vi "Point To Row.vi"(8 "error in (no error)":errorcluster, 10 "Point":T1, 11 "ListBox in":refnum<class "ListBox.lvclass">) -> (0 "error out":errorcluster, 1 "Row":i32, 2 "In Bounds?":bool, 3 "ListBox out":refnum<class "ListBox.lvclass">, 4 "In Symbol?":bool)   [LabVIEW 2015, in "ListBox.lvclass"]
doc: "Converts a pixel coordinate to a row in the coordinates of the control. This method also returns whether the point is inside the bounds of the content rectangle and whether the point is within the custom symbol of the cell.\n\nQControl Class wrapper around the <b>ListBox : Point to Row Method</b>.\n<b> </b> <b> </b>\n©2016 Q Software Innovations, LLC (QSI)\nwritten by Quentin Alldredge\nproduced in LabVIEW 2015\n\nsupport@qsoftwareinnovations.com\nwww.qsoftwareinnovations.com\n\nAll rights reserved.\n\nRedistribution and use in source and binary forms, with or without modification, are permitted provided that the following conditions are met:\n\n * Redistributions of source code must retain the above copyright notice, this list of conditions and the following disclaimer.\n * Redistributions in binary form must reproduce the above copyright notice, this list of conditions and the following disclaimer in the documentation and/or other materials provided with the distribution.\n * Neither the name of Q Software Innovations, LLC. nor the names of its contributors may be used to endorse or promote products derived from this software without specific prior written permission.\n\nTHIS SOFTWARE IS PROVIDED BY THE COPYRIGHT HOLDERS AND CONTRIBUTORS \"AS IS\" AND ANY EXPRESS OR IMPLIED WARRANTIES, INCLUDING, BUT NOT LIMITED TO, THE IMPLIED WARRANTIES OF MERCHANTABILITY AND FITNESS FOR A PARTICULAR PURPOSE ARE DISCLAIMED. IN NO EVENT SHALL THE COPYRIGHT OWNER OR CONTRIBUTORS BE LIABLE FOR ANY DIRECT, INDIRECT, INCIDENTAL, SPECIAL, EXEMPLARY, OR CONSEQUENTIAL DAMAGES (INCLUDING, BUT NOT LIMITED TO, PROCUREMENT OF SUBSTITUTE GOODS OR SERVICES; LOSS OF USE, DATA, OR PROFITS; OR BUSINESS INTERRUPTION) HOWEVER CAUSED AND ON ANY THEORY OF LIABILITY, WHETHER IN CONTRACT, STRICT LIABILITY, OR TORT (INCLUDING NEGLIGENCE OR OTHERWISE) ARISING IN ANY WAY OUT OF THE USE OF THIS SOFTWARE, EVEN IF ADVISED OF THE POSSIBILITY OF SUCH DAMAGE."
uses:
  ListBox.lvclass
  <vilib>/Utility/miscctls.llb/LVPositionTypeDef.ctl
  ListBox.lvclass/ListBox.ctl
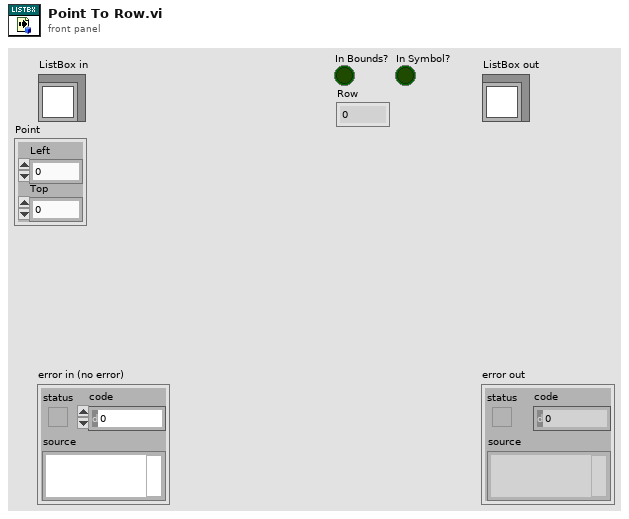
[diagram p1: front panel]
types:
  T1 = typedef "LVPositionTypeDef.ctl" = cluster{"Left":i32, "Top":i32}
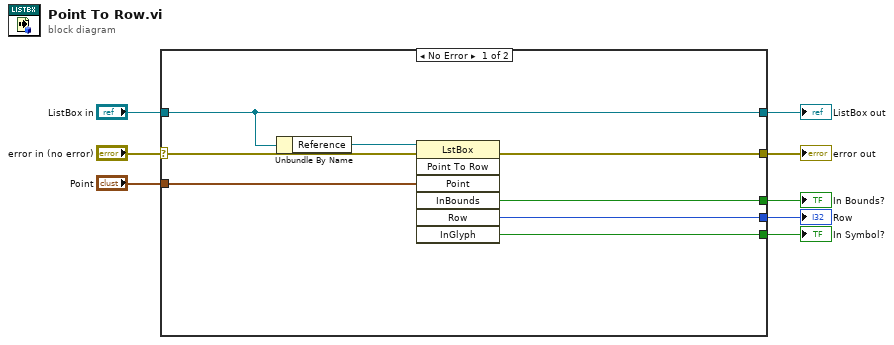
[diagram p0: block diagram]
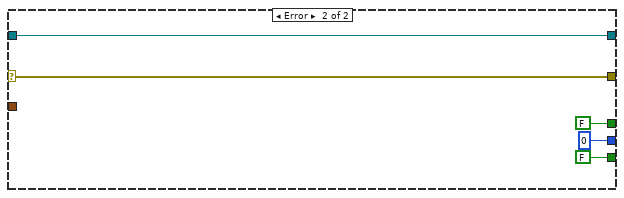
[diagram p2: hidden frame]
diagram:
  n1 = case shown="No Error" "error in (no error)" {
    selector: "error in (no error)" -> [w16 w21]
    tunnel: [w15 w21] -> w7
    tunnel: [w14 w20] -> w5
    tunnel: "ListBox in" -> [w14 w20]
    tunnel: "Point" -> [w12 _]
    tunnel: [w11 FALSE ("InBounds")] -> w3
    tunnel: [w10 0 ("Row")] -> w2
    tunnel: [w9 FALSE ("InGlyph")] -> w1
    frame No Error {
      n2 = Unbundle By Name(w14) -> ("Reference"=w13:refnum<vi>)
      n3 = invoke class="LstBox" method="Point To Row"(reference=w13, error in=w16, "Point"=w12) -> (error out=w15:errorcluster, "InBounds"=w11:bool, "Row"=w10:i32, "InGlyph"=w9:bool)  [unwired: 4 in, 3 out]
    }
    frame Error {
    }
  }
  "error out" <- w7
  "ListBox out" <- w5
  "In Bounds?" <- w3
  "Row" <- w2
  "In Symbol?" <- w1
